vi "DSA Measure Signal Amplitude and Levels 1.vi"(0 "AI Task ID In":refnum<k21>, 1 "AO Task ID In":refnum<k21>[](array[refnum]), 2 "Temperature Data In":T1, 3 "Step Delay Time has Elapsed":bool, 4 "Test Time has Elapsed":bool, 5 "error in":errorcluster, 7 "samples per channel":i32=-1, 9 "Run Mode (Manual = True)":bool) -> (10 "Load Data":bool, 14 "Task ID Cluster":T2, 15 "DSA Measurements Array":dbl[][](array[numeric]), 16 "DSA Measurements":T4, 17 "DSA Functions":T3, 18 "Temperature Data Out":T1, 19 "error out":errorcluster)   [LabVIEW 2018]
uses:
  Controls/DSA Measurements.ctl
  Controls/DSA Readings.ctl
  Controls/DSA Functions.ctl
  <vilib>/DAQmx/read.llb/DAQmx Read (Analog 1D DBL NChan 1Samp).vi
  <vilib>/DAQmx/read.llb/DAQmx Read (Analog 1D Wfm NChan NSamp).vi
  <vilib>/DAQmx/create/channels.llb/DAQmx Create Channel (AI-Temperature-Thermocouple).vi
  <vilib>/DAQmx/configure/timing.llb/DAQmx Timing (Sample Clock).vi
  <vilib>/DAQmx/miscellaneous.llb/DAQmx Fill In Error Info.vi
  <vilib>/measure/madcrms.llb/Basic Averaged DC-RMS for N Chan.vi
  <vilib>/measure/NI_MAPro.lvlib
  <resource>/objmgr/daqmx.rc
panel:
  in  "Timeout":dbl=10.0 format="%0.2f"
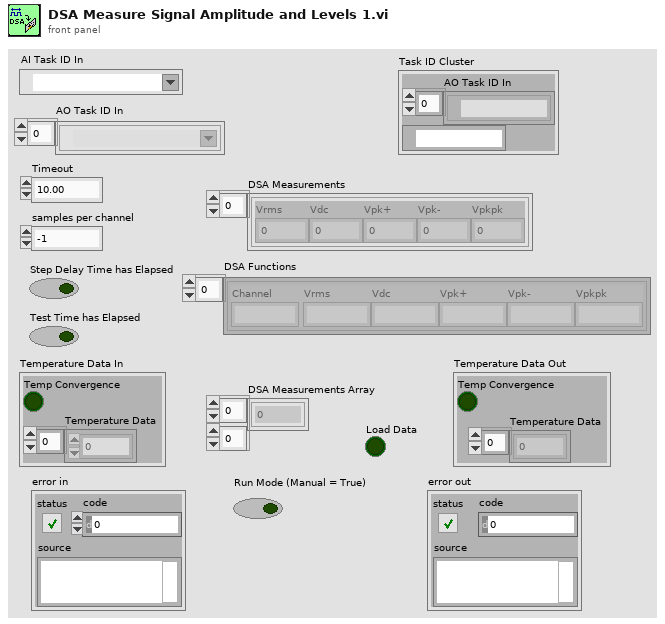
[diagram p1: front panel]
types:
  T1 = cluster{"Temp Convergence":bool, "Temperature Data":dbl[]}
  T2 = cluster{"AO Task ID In":refnum<k21>[], "task out":refnum<k21>}
  T3 = typedef "DSA Functions.ctl" = cluster{"Channel":string, "Vrms":string, "Vdc":string, "Vpk+":string, "Vpk-":string, "Vpkpk":string}[]
  T4 = typedef "DSA Measurements.ctl" = T5[]
  T5 = typedef "DSA Readings.ctl" = cluster{"Vrms":dbl, "Vdc":dbl, "Vpk+":dbl, "Vpk-":dbl, "Vpkpk":dbl}
  T6 = cluster{"[0]":string, "[1]":string, "[2]":string, "[3]":string, "[4]":string, "[5]":string}[]
  T7 = cluster{"Numeric":dbl, "Numeric":dbl, "-Peak value":dbl, "+Peak value":dbl, "Peak-Peak value":dbl}[]
  T8 = enum16{"Rectangular (none)", "Hanning", "Low side lobe"}
  T9 = cluster{"[0]":string, "[1]":string, "[2]":string, "[3]":string, "[4]":string, "[5]":string}
  T10 = cluster{dbl, "Numeric":dbl, "-Peak value":dbl, "+Peak value":dbl, "Peak-Peak value":dbl}
  T11 = cluster{"Numeric":dbl, "Numeric":dbl, "-Peak value":dbl, "+Peak value":dbl, "Peak-Peak value":dbl}
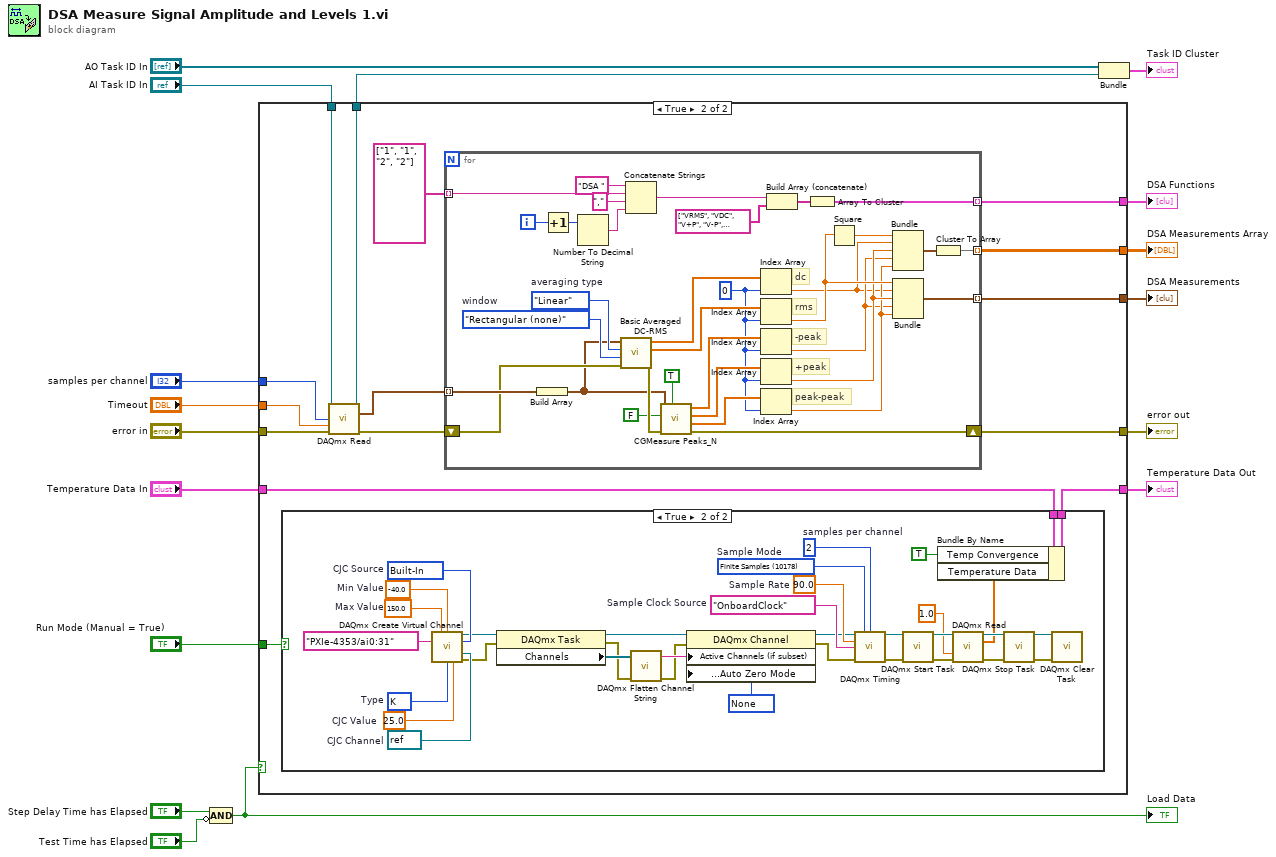
[diagram p0: block diagram]
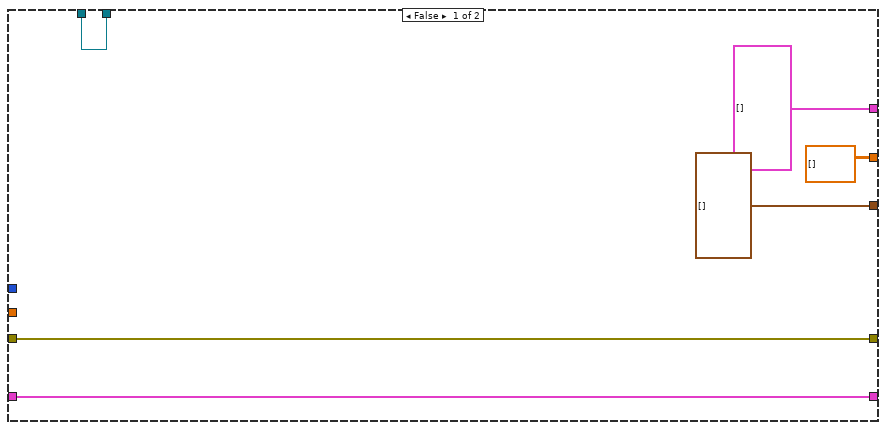
[diagram p2: hidden frame]
diagram:
  n1 = Compound Arithmetic op=AND("Step Delay Time has Elapsed", invert "Test Time has Elapsed") -> (w9:bool)
  "Load Data" <- w9
  n2 = case shown="True" w9 {
    tunnel: [T7 [] w38] -> w17
    tunnel: "Timeout" -> [_ w37]
    tunnel: [dbl[][] [] w36] -> w15
    tunnel: "error in" -> [w22 w35]
    tunnel: "AI Task ID In" -> [w23 w34]
    tunnel: [w22 w33] -> w4
    tunnel: [T6 [] w32] -> w14
    tunnel: "samples per channel" -> [_ w31]
    tunnel: [w23 w30] -> w5
    tunnel: [w18 w25] -> w3
    tunnel: "Temperature Data In" -> [w18 w26]
    tunnel: "Run Mode (Manual = True)" -> [_ w24]
    frame False {
    }
    frame True {
      n3 = case shown="True" w24 {
        tunnel: w26 -> [w39 w73]
        tunnel: [w39 w72] -> w25
        frame False {
        }
        frame True {
          w41 = 2  # samples per channel
          w47 = 10230 items=["None"=10230, "Once"=10244, "Every Sample"=10164] ("Auto Zero Mode")
          w65 = refnum<k21> refnum  # CJC Channel
          w60 = 10200 items=["Built-In"=10200, "Constant Value"=10116, "Channel"=10113]  # CJC Source
          w61 = -40.0  # Min Value
          w62 = 150.0  # Max Value
          w64 = 25.0  # CJC Value
          w63 = 10073 items=["J"=10072, "K"=10073, "N"=10077, "R"=10082, "S"=10085, "T"=10086, "B"=10047, "E"=10055]  # Type
          w57 = 90.0  # Sample Rate
          w58 = tag "OnboardClock"  # Sample Clock Source
          w59 = 10178 items=["Finite Samples"=10178, "Continuous Samples"=10123, "Hardware Timed Single Point"=12522]  # Sample Mode
          n4 = call-poly <vilib>:"DAQmx Create Virtual Channel.vi"("maximum value"=w62, "minimum value"=w61, "physical channels"=tag "PXIe-4353/ai0:31" ("Physical Channel"), "cjc source"=w60, "cjc channel"=w65, "thermocouple type"=w63, "cjc value"=w64) -> ("task out"=w56:refnum<k21>, "error out"=w54:errorcluster)  [unwired: 7 in]
          n5 = property class="DAQmx Task"(reference=w56, error in=w54) -> (reference out=w52:refnum<k21>, error out=w49:errorcluster, "Channels"=w51:refnum<k21>[])
          n6 = call <vilib>:"DAQmx Flatten Channel String.vi"("names in"=w51, "error in"=w49) -> ("names out"=w50:string, "error out"=w48:errorcluster)  [unwired: 12 in]
          n7 = property class="DAQmx Channel"(reference=w52, error in=w48, "Active Channels (if subset)"=w50, "Analog Input:General Properties:Advanced:High Accuracy Settings:Auto Zero Mode"=w47) -> (reference out=w55:refnum<k21>, error out=w53:errorcluster)
          n8 = call-poly <vilib>:"DAQmx Timing.vi"("task/channels in"=w55, "sample mode"=w59, "samples per channel"=w41, "rate"=w57, "source"=w58, "error in"=w53) -> ("task out"=w66:refnum<k21>, "error out"=w46:errorcluster)  [unwired: 8 in]
          n9 = call <vilib>:"DAQmx Start Task.vi"("task/channels in"=w66, "error in"=w46) -> ("task out"=w44:refnum<k21>, "error out"=w43:errorcluster)  [unwired: 12 in]
          n10 = call-poly <vilib>:"DAQmx Read.vi"("task/channels in"=w44, "timeout"=1.0, "error in"=w43) -> ("task out"=w68:refnum<k21>, "data"=w40:dbl[], "error out"=w67:errorcluster)  [unwired: 10 in]
          n11 = Bundle By Name(cluster=w73, "Temp Convergence"=TRUE, "Temperature Data"=w40) -> (w72:T1)
          n12 = call <vilib>:"DAQmx Stop Task.vi"("task/channels in"=w68, "error in"=w67) -> ("task out"=w70:refnum<k21>, "error out"=w69:errorcluster)  [unwired: 12 in]
          n13 = call <vilib>:"DAQmx Clear Task.vi"("task in"=w70, "error in"=w69) -> ()  [unwired: 13 in, 1 out]
        }
      }
      n14 = call-poly <vilib>:"DAQmx Read.vi"("task/channels in"=w34, "number of samples per channel"=w31, "timeout"=w37, "error in"=w35) -> ("task out"=w30:refnum<k21>, "data"=w29:waveform(dbl)[], "error out"=w28:errorcluster)  [unwired: 9 in]
      n15 = for {
        tunnel: w29 -> [w107] mode=indexing
        shift-right: [w105] -> w33
        shift-left: w28 -> [w106]
        tunnel: [w94] -> w36 mode=indexing
        tunnel: [w93] -> w38 mode=indexing
        tunnel: [w83] -> w32 mode=indexing
        tunnel: string[] ["1", "1", "2", "2"] ("Array") -> [w82] mode=indexing
        i -> [w84]
        w92 = 0 ("index")
        w102 = T8."Rectangular (none)"  # window
        w103 = enum16{"Linear", "Exponential"}."Linear"  # averaging type
        # "+peak"
        # "peak-peak"
        # "-peak"
        # "rms"
        # "dc"
        n16 = Build Array(w107) -> (w91:waveform(dbl)[])
        n17 = Increment(x=w84) -> (x+1=w87:i32)
        n18 = Number To Decimal String(number=w87) -> (decimal integer string=w88:string)  [unwired: 1 in]
        n19 = call-poly <vilib>:"Basic Averaged DC-RMS.vi"("error in (no error)"=w106, "window"=w102, "averaging type"=w103, "signals in"=w91) -> ("error out"=w104:errorcluster, "RMS values"=w99:dbl[], "DC values"=w100:dbl[])  [unwired: 4 in, 1 out]
        n20 = Concatenate Strings("DSA " ("string"), w82, "," ("string"), w88) -> (w89:string)
        n21 = call <vilib>:"CGMeasure Peaks_N.vi"("reset"=TRUE, "error in (no error)"=w104, "hold"=FALSE ("hold peaks"), "signals in"=w91) -> ("error out"=w105:errorcluster, "Peak-Peak values"=w96:dbl[], "-Peak values"=w97:dbl[], "+Peak values"=w98:dbl[])  [unwired: 4 in]
        n22 = Index Array(array=w100, index=w92) -> (element=w76:dbl)
        n23 = Index Array(array=w99, index=w92) -> (element=w80:dbl)
        n24 = Index Array(array=w98, index=w92) -> (element=w77:dbl)
        n25 = Index Array(array=w97, index=w92) -> (element=w79:dbl)
        n26 = Index Array(array=w96, index=w92) -> (element=w78:dbl)
        n27 = Build Array (concatenate)(w89, string[] ["VRMS", "VDC", "V+P", "V-P", "VPkPk"] ("DSA Functions")) -> (w90:string[])
        n28 = Array To Cluster(array=w90) -> (cluster=w83:T9)
        n29 = Square(x=w80) -> (x^2=w74:dbl)
        n30 = Bundle(w74, "Numeric"=w76, "-Peak value"=w79, "+Peak value"=w77, "Peak-Peak value"=w78) -> (w75:T10)  [unwired: 1 in]
        n31 = Bundle("Numeric"=w80, "Numeric"=w76, "-Peak value"=w79, "+Peak value"=w77, "Peak-Peak value"=w78) -> (w93:T11)  [unwired: 1 in]
        n32 = Cluster To Array(cluster=w75) -> (array=w94:dbl[])
      }
    }
  }
  "DSA Measurements" <- w17
  "DSA Measurements Array" <- w15
  "DSA Functions" <- w14
  "error out" <- w4
  "Temperature Data Out" <- w3
  n33 = Bundle("AO Task ID In"="AO Task ID In", "task out"=w5) -> (→"Task ID Cluster":T2)  [unwired: 1 in]
